vi "helper - polar plot labels nautical degrees.vi"(0 "grid measurements":T2 {"end angle" format="%0.2f"; "start angle" format="%0.2f"; "scale factors"."b" format="%0.2f"; "scale factors"."a" format="%0.2f"}, 4 "picture":picture, 5 "desired font(Application)":T3(ring)=enum."Application Font", 6 "[user-specified font]":T4) -> (7 "new picture":picture)   [LabVIEW 2011]
panel:
  in  "label justification":T1(array[cluster])=[{"horizontal"=enum."left", "vertical"=enum."center"}, {"horizontal"=enum."center", "vertical"=enum."bottom"}, {"horizontal"=enum."right", "vertical"=enum."center"}, {"horizontal"=enum."center", "vertical"=enum."top"}]
  in  "axis labels":string[](array[string])=["", "0=360", "270", "180"]
  # "These arrays are\nused to decide \nwhat the text for\nthe labels is."
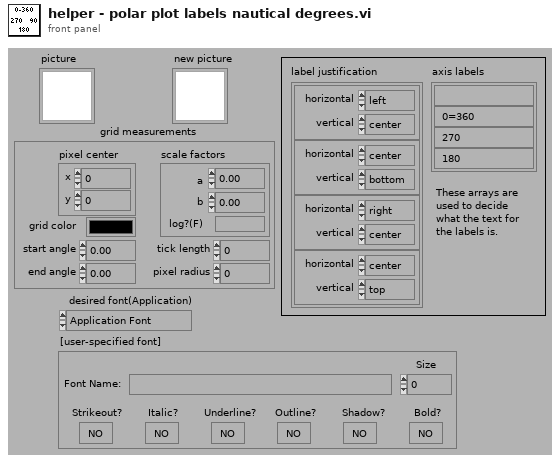
[diagram p1: front panel]
types:
  T1 = cluster{"horizontal":enum16{"left", "center", "right"}, "vertical":enum16{"top", "center", "bottom"}}[]
  T2 = cluster{"pixel center":cluster{"x":i16, "y":i16}, "scale factors":cluster{"a":dbl, "b":dbl, "log?(F)":bool}, "grid color":u32, "start angle":dbl, "end angle":dbl, "tick length":i16, "pixel radius":i32}
  T3 = enum16{"User-specified Font", "Application Font", "System Font", "Dialog Font"}
  T4 = cluster{"Font Name:":string, "Size":i16, "Strikeout?":bool, "Italic?":bool, "Underline?":bool, "Outline?":bool, "Shadow?":bool, "Bold?":bool}
  T5 = cluster{"horizontal":enum16{"left", "center", "right"}, "vertical":enum16{"top", "center", "bottom"}}
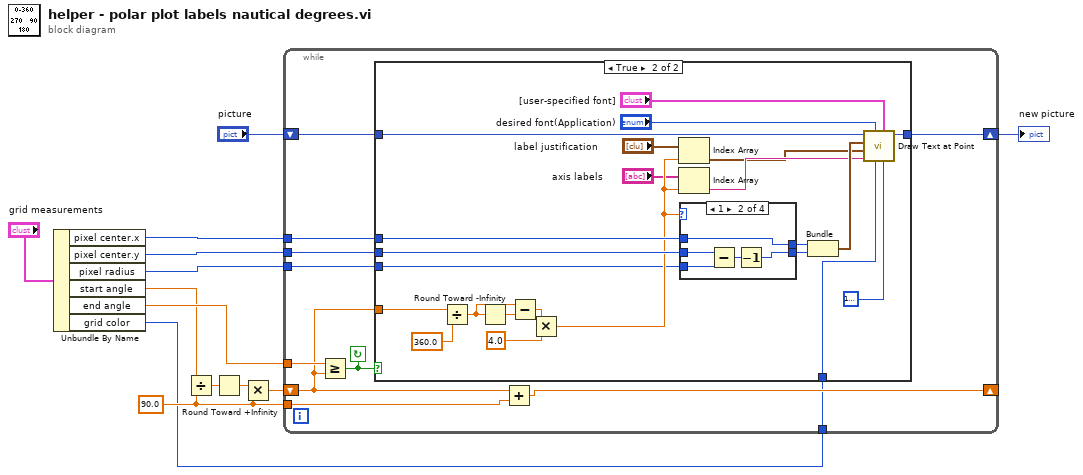
[diagram p0: block diagram]
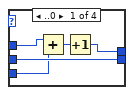
[diagram p3: hidden frame]
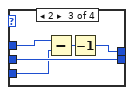
[diagram p4: hidden frame]
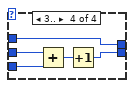
[diagram p5: hidden frame]
diagram:
  w7 = 90.0
  n1 = Unbundle By Name("grid measurements") -> ("pixel center.x"=w2:i16, "pixel center.y"=w3:i16, "pixel radius"=w4:i32, "start angle"=w5:dbl, "end angle"=w6:dbl, "grid color"=w1:u32)
  n2 = Divide(x=w5, y=w7) -> (x/y=w10:dbl)
  n3 = Round Toward +Infinity(x=w10) -> (ceil(x): smallest int >= x=w9:dbl)
  n4 = Multiply(x=w9, y=w7) -> (x*y=w8:dbl)
  n5 = while {
    tunnel: w2 -> [w15]
    tunnel: w3 -> [w16]
    tunnel: w4 -> [w17]
    shift-left: "picture" -> [w18]
    shift-right: [w19] -> w12
    tunnel: w6 -> [w23]
    tunnel: w7 -> [w24]
    shift-left: w8 -> [w20]
    shift-right: [w22] -> _
    tunnel: w1 -> [w14]
    stop <- w21 continue-if-true
    n6 = Greater Or Equal?(x=w23, y=w20) -> (x >= y?=w21:bool)
    n7 = case shown="True" w21 {
      tunnel: w20 -> [_ w43]
      tunnel: [w25 w38] -> w19
      tunnel: w18 -> [w25 w37]
      tunnel: w17 -> [_ w27]
      tunnel: w16 -> [_ w36]
      tunnel: w15 -> [_ w35]
      tunnel: w14 -> [_ w26]
      frame False {
      }
      frame True {
        n8 = Divide(x=w43, y=360.0) -> (x/y=w46:dbl)
        n9 = Round Toward -Infinity(1:w46) -> (0:w45:dbl)
        n10 = Subtract(x=w46, y=w45) -> (x-y=w47:dbl)
        n11 = Multiply(x=w47, y=4.0) -> (x*y=w32:dbl)
        n12 = Index Array(array="label justification", index=w32) -> (element=w28:T5)
        n13 = Index Array(array="axis labels", index=w32) -> (element=w29:string)
        n14 = case shown="1" w32 {
          tunnel: w35 -> [w51 w58 w63 w68]
          tunnel: w36 -> [w53 w57 w61 w67]
          tunnel: [w50 w58 w60 w68] -> w39
          tunnel: [w53 w55 w61 w65] -> w40
          tunnel: w27 -> [w49 w54 w59 w64]
          frame ..0 {
            n15 = Add(x=w51, y=w49) -> (x+y=w52:i32)
            n16 = Increment(x=w52) -> (x+1=w50:i32)
          }
          frame 1 {
            n17 = Subtract(x=w57, y=w54) -> (x-y=w56:i32)
            n18 = Decrement(x=w56) -> (x-1=w55:i32)
          }
          frame 2 {
            n19 = Subtract(x=w63, y=w59) -> (x-y=w62:i32)
            n20 = Decrement(x=w62) -> (x-1=w60:i32)
          }
          frame 3.. {
            n21 = Add(x=w67, y=w64) -> (x+y=w66:i32)
            n22 = Increment(x=w66) -> (x+1=w65:i32)
          }
        }
        n23 = Bundle("x"=w39, "y"=w40) -> (w41:cluster{"x":i32, "y":i32})  [unwired: 1 in]
        n24 = call <vilib>:"Draw Text at Point.vi"("BG color(transparent)"=u32 16777216, "[user-specified font]"="[user-specified font]", "text color(black)"=w26, "desired font(Application)"="desired font(Application)", "text"=w29, "alignment(left, top)"=w28, "origin"=w41, "picture"=w37) -> ("new picture"=w38:picture)  [unwired: 2 in, 1 out]
      }
    }
    n25 = Add(x=w20, y=w24) -> (x+y=w22:dbl)
  }
  "new picture" <- w12
